vi "comm flow control.vi"(4 "XON Character":u8=11, 6 "XOFF Character":u8=13, 8 "error in (no error)":errorcluster, 10 "Flow Control":u16(ring) items=["None"=0, "XON/XOFF"=1, "RTS/CTS"=2, "DTR/DSR"=4], 11 "Comm Handle":u64) -> (0 "error out":errorcluster, 3 "dup Comm Handle":u64)   [LabVIEW 2021, in "lvserial.lvlib"]
doc: "Sets the flow control mode."
uses:
  lvserial.lvlib
  lvserial.dll
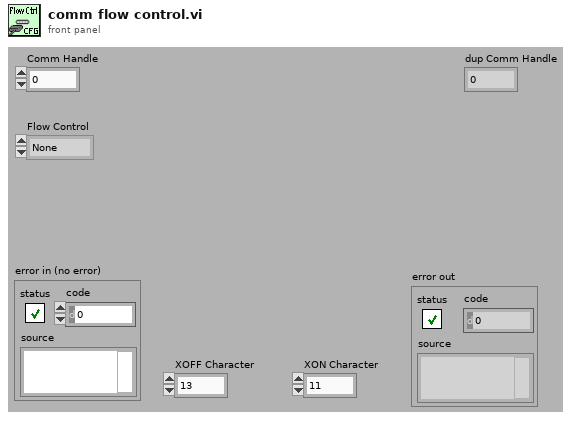
[diagram p1: front panel]
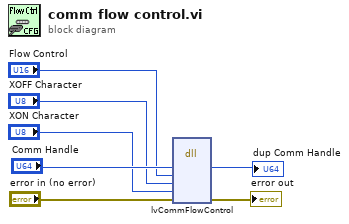
[diagram p0: block diagram]
diagram:
  n1 = dll-call lib="lvserial.dll" fn="lvCommFlowControl"("hComm"="Comm Handle", "usFlowControl"="Flow Control", "ucXOFFCharacter"="XOFF Character", "ucXONCharacter"="XON Character", "error"="error in (no error)") -> ("hComm"=→"dup Comm Handle":u64, "error"=→"error out":errorcluster)  [unwired: 6 in, 3 out]
